vi "_Get Simulation Data.vi"(4 "SimulationMass":dbl[](array[numeric]), 5 "ErrorIn":errorcluster, 6 "SimulationSpectrum":i32[](array[numeric]), 7 "CurrentExpt#":i32, 8 "CurrentRetTime":i32) -> (0 "ErrorOut":errorcluster, 1 "DataArray":i32[](array[numeric]), 2 "NextExpt#":i32, 3 "NextRetTime":i32)   [LabVIEW 2015]
uses:
  Configuration/_Global Configuration.vi
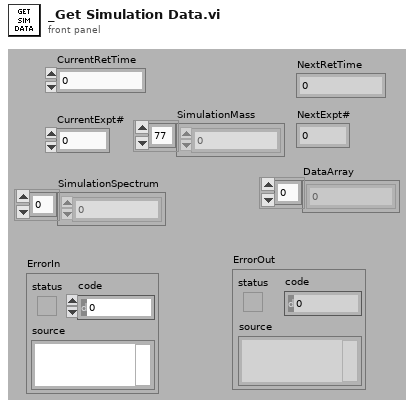
[diagram p1: front panel]
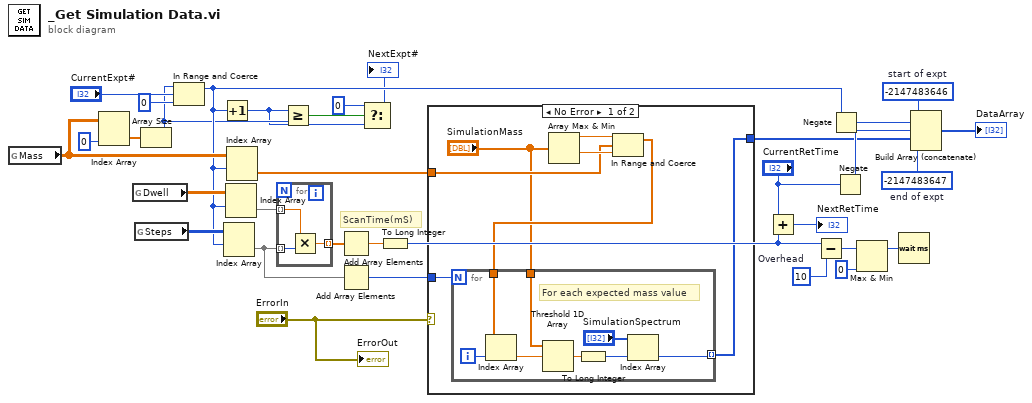
[diagram p0: block diagram]
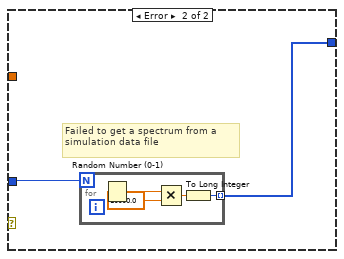
[diagram p2: hidden frame]
diagram:
  w20 = 10  # Overhead
  w27 = -2147483646  # start of expt
  w26 = -2147483647  # end of expt
  # "ScanTime(mS)"
  n1 = global read "_Global Configuration.vi" "Mass"() -> (w16:dbl[][])
  n2 = Index Array(array=w16, index (col)=0 ("disabled index (col)")) -> (element=w14:dbl[])  [unwired: 1 in]
  n3 = global read "_Global Configuration.vi" "Dwell"() -> (w33:dbl[][])
  n4 = global read "_Global Configuration.vi" "Steps"() -> (w32:i32[][])
  n5 = Array Size(array=w14) -> (size(s)=w10:i32)
  n6 = In Range and Coerce(upper limit=w10, x="CurrentExpt#", lower limit=0) -> (coerced(x)=w11:i32)  [unwired: 1 out]
  n7 = Increment(x=w11) -> (x+1=w8:i32)
  n8 = Index Array(array=w32, index (row)=w11) -> (element=w3:i32[])  [unwired: 1 in]
  n9 = Index Array(array=w33, index (row)=w11) -> (element=w31:dbl[])  [unwired: 1 in]
  n10 = Index Array(array=w16, index (row)=w11) -> (element=w28:dbl[])  [unwired: 1 in]
  n11 = for {
    tunnel: w31 -> [w36] mode=indexing
    tunnel: w3 -> [w35] mode=indexing
    tunnel: [w34] -> w30 mode=indexing
    n12 = Multiply(x=w36, y=w35) -> (x*y=w34:dbl)
  }
  n13 = Greater Or Equal?(x=w8, y=w10) -> (x >= y?=w9:bool)
  n14 = Add Array Elements(numeric array=w30) -> (sum=w29:dbl)
  n15 = Add Array Elements(numeric array=w3) -> (sum=w4:i32)
  n16 = Select(t=0, s=w9, f=w8) -> (s? t:f=→"NextExpt#":i32)
  n17 = To Long Integer(number=w29) -> (32bit integer=w5:i32)
  n18 = case shown="No Error" "ErrorIn" {
    tunnel: w28 -> [w40 _]
    tunnel: w4 -> [w43 w53]
    tunnel: [w37 w52] -> w1
    frame No Error {
      n19 = Array Max & Min(array="SimulationMass") -> (max value=w42:dbl, min value=w41:dbl)  [unwired: 2 out]
      n20 = In Range and Coerce(upper limit=w42, x=w40, lower limit=w41) -> (coerced(x)=w39:dbl[])  [unwired: 1 out]
      n21 = for {
        N: w43 -> [_]
        tunnel: w39 -> [w48]
        tunnel: "SimulationMass" -> [w47]
        tunnel: [w44] -> w37 mode=indexing
        i -> [w51]
        # "For each expected mass value"
        n22 = Index Array(array=w48, index=w51) -> (element=w49:dbl)
        n23 = Threshold 1D Array(2:w49, 3:w47) -> (0:w50:dbl)  [unwired: 1 in]
        n24 = To Long Integer(number=w50) -> (32bit integer=w46:i32)
        n25 = Index Array(array="SimulationSpectrum", index=w46) -> (element=w44:i32)
      }
    }
    frame Error {
      # "Failed to get a spectrum from a simulation data file"
      n26 = for {
        N: w53 -> [_]
        tunnel: [w54] -> w52 mode=indexing
        n27 = Random Number (0-1)() -> (number: 0 to 1=w57:dbl)
        n28 = Multiply(x=w57, y=10000.0) -> (x*y=w55:dbl)
        n29 = To Long Integer(number=w55) -> (32bit integer=w54:i32)
      }
    }
  }
  n30 = Add(x="CurrentRetTime", y=w5) -> (x+y=→"NextRetTime":i32)
  n31 = Subtract(x=w5, y=w20) -> (x-y=w19:i32)
  n32 = Negate(x=w11) -> (-x=w24:i32)
  n33 = Negate(x="CurrentRetTime") -> (-x=w23:i32)
  n34 = Max & Min(x=w19, y=0) -> (max(x,y)=w17:i32)  [unwired: 1 out]
  n35 = Wait (ms)(milliseconds to wait=w17) -> ()  [unwired: 1 out]
  n36 = Build Array (concatenate)(w27, w24, w23, w1, w26) -> (→"DataArray":i32[])
  "ErrorOut" <- "ErrorIn"
